vi "hmi_get_joystick_data.vi"() -> (3 "UserData":T1)   [LabVIEW 2011]
uses:
  user_data.ctl
  user_buttons_dualaction.ctl
  user_buttons_360.ctl
  <vilib>/Rock Robotics/WPI/Joystick/WPI_JoystickDevRef.ctl
  <vilib>/Rock Robotics/WPI/Joystick/WPI_JoystickDeviceEnum.ctl
  script/Auto_Conf.vi
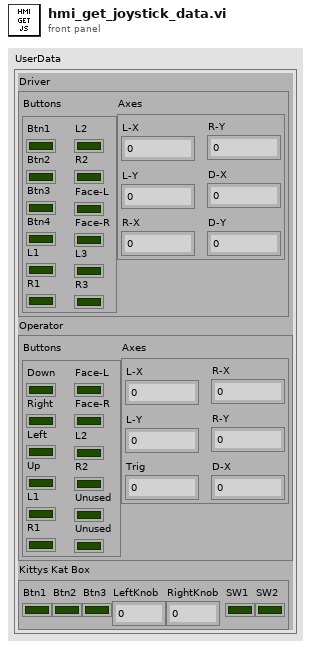
[diagram p1: front panel]
types:
  T1 = typedef "user_data.ctl" = cluster{"Driver":cluster{"Buttons":T2, "Axes":cluster{"L-X":dbl, "L-Y":dbl, "R-X":dbl, "R-Y":dbl, "D-X":dbl, "D-Y":dbl}}, "Operator":cluster{"Buttons":T3, "Axes":cluster{"L-X":dbl, "L-Y":dbl, "Trig":dbl, "R-X":dbl, "R-Y":dbl, "D-X":dbl}}, "Kittys Kat Box":cluster{"Btn1":bool, "Btn2":bool, "Btn3":bool, "LeftKnob":dbl, "RightKnob":dbl, "SW1":bool, "SW2":bool}}
  T2 = typedef "user_buttons_dualaction.ctl" = cluster{"Btn1":bool, "Btn2":bool, "Btn3":bool, "Btn4":bool, "L1":bool, "R1":bool, "L2":bool, "R2":bool, "Face-L":bool, "Face-R":bool, "L3":bool, "R3":bool}
  T3 = typedef "user_buttons_360.ctl" = cluster{"Down":bool, "Right":bool, "Left":bool, "Up":bool, "L1":bool, "R1":bool, "Face-L":bool, "Face-R":bool, "L2":bool, "R2":bool, "Unused":bool, "Unused":bool}
  T4 = typedef "WPI_JoystickDevRef.ctl" = cluster{"Device":T5}
  T5 = typedef "WPI_JoystickDeviceEnum.ctl" = enum16{"USB 1", "USB 2", "USB 3", "USB 4", "Kinect 1", "Kinect 2"}
  T6 = typedef "WPI_JoystickButtonState.ctl" = cluster{"Button 1":bool, "Button 2":bool, "Button 3":bool, "Button 4":bool, "Button 5":bool, "Button 6":bool, "Button 7":bool, "Button 8":bool, "Button 9":bool, "Button 10":bool, "Button 11":bool, "Button 12":bool}
  T7 = cluster{"axis 1 (x)":dbl, "axis 2 (y)":dbl, "axis 3 (throttle)":dbl, "axis 4":dbl, "axis 5":dbl, "axis 6":dbl}
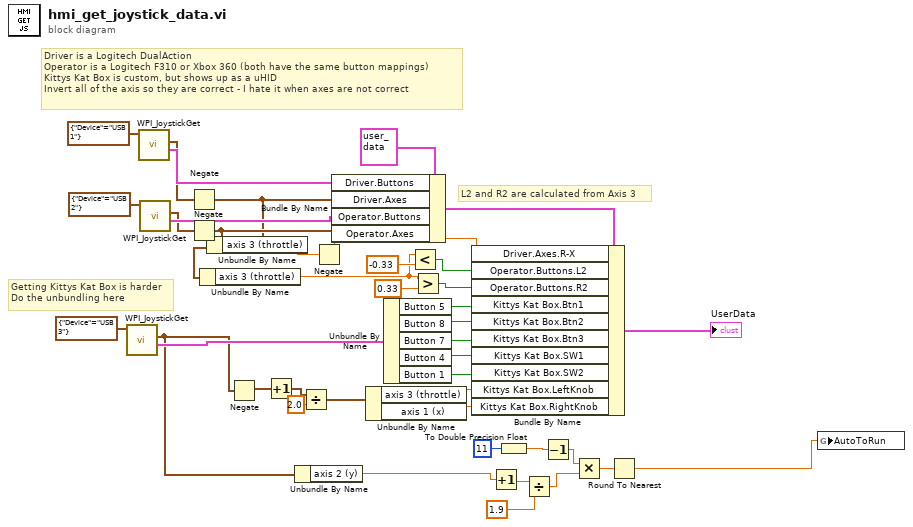
[diagram p0: block diagram]
diagram:
  # "L2 and R2 are calculated from Axis 3"
  # "Driver is a Logitech DualAction\nOperator is a Logitech F310 or Xbox 360 (both have the same button mappings)\nKittys Kat Box is custom, but shows up as a uHID\nInvert all of the axis so they are correct - I hate it when axes are not correct"
  # "Getting Kittys Kat Box is harder\nDo the unbundling here"
  n1 = call <vilib>:"WPI_JoystickGet.vi"("JoystickDevRef"=T4 {"Device"=enum."USB 3"}) -> ("Buttons"=w37:T6, "Axes"=w10:T7)  [unwired: 4 in, 1 out]
  n2 = call <vilib>:"WPI_JoystickGet.vi"("JoystickDevRef"=T4 {"Device"=enum."USB 1"}) -> ("Buttons"=w35:T6, "Axes"=w22:T7)  [unwired: 4 in, 1 out]
  n3 = call <vilib>:"WPI_JoystickGet.vi"("JoystickDevRef"=T4 {"Device"=enum."USB 2"}) -> ("Buttons"=w41:T6, "Axes"=w21:T7)  [unwired: 4 in, 1 out]
  n4 = Negate(x=w22) -> (-x=w19:T7)
  n5 = Negate(x=w21) -> (-x=w20:T7)
  n6 = Unbundle By Name(w20) -> ("axis 3 (throttle)"=w25:dbl)
  n7 = Unbundle By Name(w19) -> ("axis 3 (throttle)"=w18:dbl)
  n8 = Negate(x=w10) -> (-x=w16:T7)
  n9 = Increment(x=w16) -> (x+1=w14:T7)
  n10 = Unbundle By Name(w10) -> ("axis 2 (y)"=w2:dbl)
  n11 = Divide(x=w14, y=2.0) -> (x/y=w13:T7)
  n12 = Negate(x=w18) -> (-x=w17:dbl)
  n13 = Bundle By Name(cluster=T1 {"Driver"={"Buttons"={"Btn1"=FALSE, "Btn2"=FALSE, "Btn3"=FALSE, "Btn4"=FALSE, "L1"=FALSE, "R1"=FALSE, "L2"=FALSE, "R2"=FALSE, "Face-L"=FALSE, "Face-R"=FALSE, "L3"=FALSE, "R3"=FALSE}, "Axes"={"L-X"=0.0, "L-Y"=0.0, "R-X"=0.0, "R-Y"=0.0, "D-X"=0.0, "D-Y"=0.0}}, "Operator"={"Buttons"={"Down"=FALSE, "Right"=FALSE, "Left"=FALSE, "Up"=FALSE, "L1"=FALSE, "R1"=FALSE, "Face-L"=FALSE, "Face-R"=FALSE, "L2"=FALSE, "R2"=FALSE, "Unused"=FALSE, "Unused"=FALSE}, "Axes"={"L-X"=0.0, "L-Y"=0.0, "Trig"=0.0, "R-X"=0.0, "R-Y"=0.0, "D-X"=0.0}}, "Kittys Kat Box"={"Btn1"=FALSE, "Btn2"=FALSE, "Btn3"=FALSE, "LeftKnob"=0.0, "RightKnob"=0.0, "SW1"=FALSE, "SW2"=FALSE}} ("UserData"), "Driver.Buttons"=w35, "Driver.Axes"=w19, "Operator.Buttons"=w41, "Operator.Axes"=w20) -> (w34:T1)
  n14 = Unbundle By Name(w13) -> ("axis 3 (throttle)"=w12:dbl, "axis 1 (x)"=w11:dbl)
  n15 = Unbundle By Name(w37) -> ("Button 5"=w32:bool, "Button 8"=w31:bool, "Button 7"=w30:bool, "Button 4"=w29:bool, "Button 1"=w28:bool)
  n16 = Less?(x=w25, y=-0.33) -> (x < y?=w27:bool)
  n17 = Greater?(x=w25, y=0.33) -> (0:w24:bool)
  n18 = Bundle By Name(cluster=w34, "Driver.Axes.R-X"=w17, "Operator.Buttons.L2"=w27, "Operator.Buttons.R2"=w24, "Kittys Kat Box.Btn1"=w32, "Kittys Kat Box.Btn2"=w31, "Kittys Kat Box.Btn3"=w30, "Kittys Kat Box.SW1"=w29, "Kittys Kat Box.SW2"=w28, "Kittys Kat Box.LeftKnob"=w12, "Kittys Kat Box.RightKnob"=w11) -> (→"UserData":T1)
  n19 = Increment(x=w2) -> (x+1=w8:dbl)
  n20 = To Double Precision Float(number=11) -> (double precision float=w9:dbl)
  n21 = Divide(x=w8, y=1.9) -> (x/y=w4:dbl)
  n22 = Decrement(x=w9) -> (x-1=w5:dbl)
  n23 = Multiply(x=w5, y=w4) -> (x*y=w6:dbl)
  n24 = Round To Nearest(number=w6) -> (nearest integer value=w1:dbl)
  n25 = global write "Auto_Conf.vi" "AutoToRun"(w1) -> ()
